vi "Read fpgaClockSpeed_Hz.vi"(8 "error in (no error)":errorcluster, 11 "LoopConfigInternal in":refnum<class "LoopInternalConfig.lvclass">) -> (0 "error out":errorcluster, 2 "fpgaClockSpeed_Hz":dbl, 3 "LoopConfigInternal out":refnum<class "LoopInternalConfig.lvclass">)   [LabVIEW 2013, in "ComponentData.lvlib" / "LoopInternalConfig.lvclass"]
uses:
  <userlib>/Common/Component/Application/RT/ComponentData/ConfigurationHandler/LoopInternalConfig/LoopInternalConfig.lvclass
  <userlib>/Common/Component/Application/RT/ComponentData/ConfigurationHandler/LoopInternalConfig/LoopInternalConfig.lvclass/LoopInternalConfig.ctl
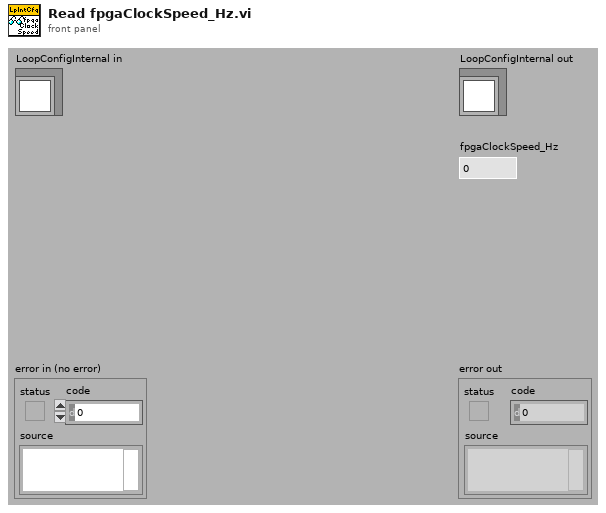
[diagram p1: front panel]
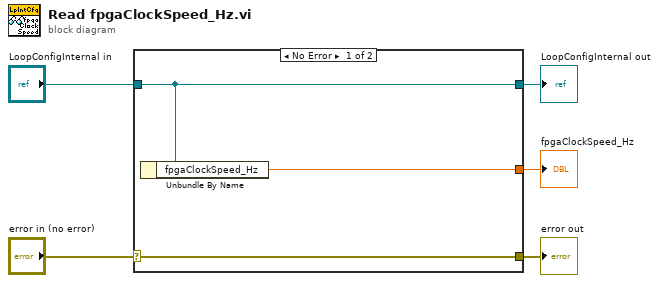
[diagram p0: block diagram]
diagram:
  n1 = case shown="No Error" "error in (no error)" {
    selector: "error in (no error)" -> [w8 w9]
    tunnel: [w8 w9] -> w4
    tunnel: [w7 w10] -> w2
    tunnel: "LoopConfigInternal in" -> [w7 w10]
    tunnel: [w6 _] -> w1
    frame No Error {
      n2 = Unbundle By Name(w7) -> ("fpgaClockSpeed_Hz"=w6:dbl)
    }
    frame Error {
    }
  }
  "error out" <- w4
  "LoopConfigInternal out" <- w2
  "fpgaClockSpeed_Hz" <- w1
